vi "Serial_read.vi"() -> ()   [LabVIEW 2016]
uses:
  Program Files (x86)/National Instruments/LabVIEW 2016/examples/Instrument IO/Serial/support/Serial - Settings.ctl
  Program Files (x86)/National Instruments/LabVIEW 2016/examples/Instrument IO/Serial/support/Serial - XON-XOFF Characters.ctl
  Program Files (x86)/National Instruments/LabVIEW 2016/examples/Instrument IO/Serial/support/Serial - ASCII Characters.ctl
  <vilib>/Instr/_visa.llb/VISA Configure Serial Port (Instr).vi
  <vilib>/Utility/file.llb/Write Delimited Spreadsheet (DBL).vi
panel:
  out "element":dbl
  out "error out":errorcluster
  out "Serial Settings:Number of Bytes at Serial Port":u32
  out "Byte array has been sent":u8[](array[numeric])
  in  "Payload  Byte to be sent":u8[](array[numeric])
  in  "Type of Message to be sent":T1(ring)
  in  "MCU Address to be sent":string(combo)
  in  "Save":bool
  out "Waveform Chart 2":dbl(graph)
  out "Thermometer":dbl(slide) scale=0.0..100.0
  out "Waveform Chart":dynamicdata(graph)
  out "Extracted Numbers":dbl[](array[numeric]) format="%#.6g"
  in  "Stop":bool
  out "String":string
  in  "Termination Character":u8=10 format="%.0x"
  in  "End Write on Termination Character?":bool=TRUE
  in  "VISA resource name":refnum<visa-resource-name>="COM1"
  in  "XON/XOFF Characters":T2={"XON"=enum."DC1", "XOFF"=enum."DC3"}
  in  "Serial Settings":T4={"baud rate"=9600, "data bits"=8, "parity"=enum."None", "stop bits"=10, "flow control"=0} {"flow control" items=["None"=0, "XON/XOFF"=1, "RTS/CTS"=2, "DTR/DSR"=4]; "stop bits" items=["1.0"=10, "1.5"=15, "2.0"=20]; "data bits" min=5 max=8 step=1; "baud rate" items=["75"=75, "110"=110, "134"=134, "150"=150, "300"=300, "600"=600, "1200"=1200, "1800"=1800, "2400"=2400, "4800"=4800, "7200"=7200, "9600"=9600, "14400"=14400, "19200"=19200, "28800"=28800, "38400"=38400, "56000"=56000, "57600"=57600, "115200"=115200, "128000"=128000, "230400"=230400]}
  in  "End Read on Termination Character?":bool=TRUE
  out "Response":string
  in  "Read Count":u32=1000
  in  "Read":bool
  in  "Write":bool
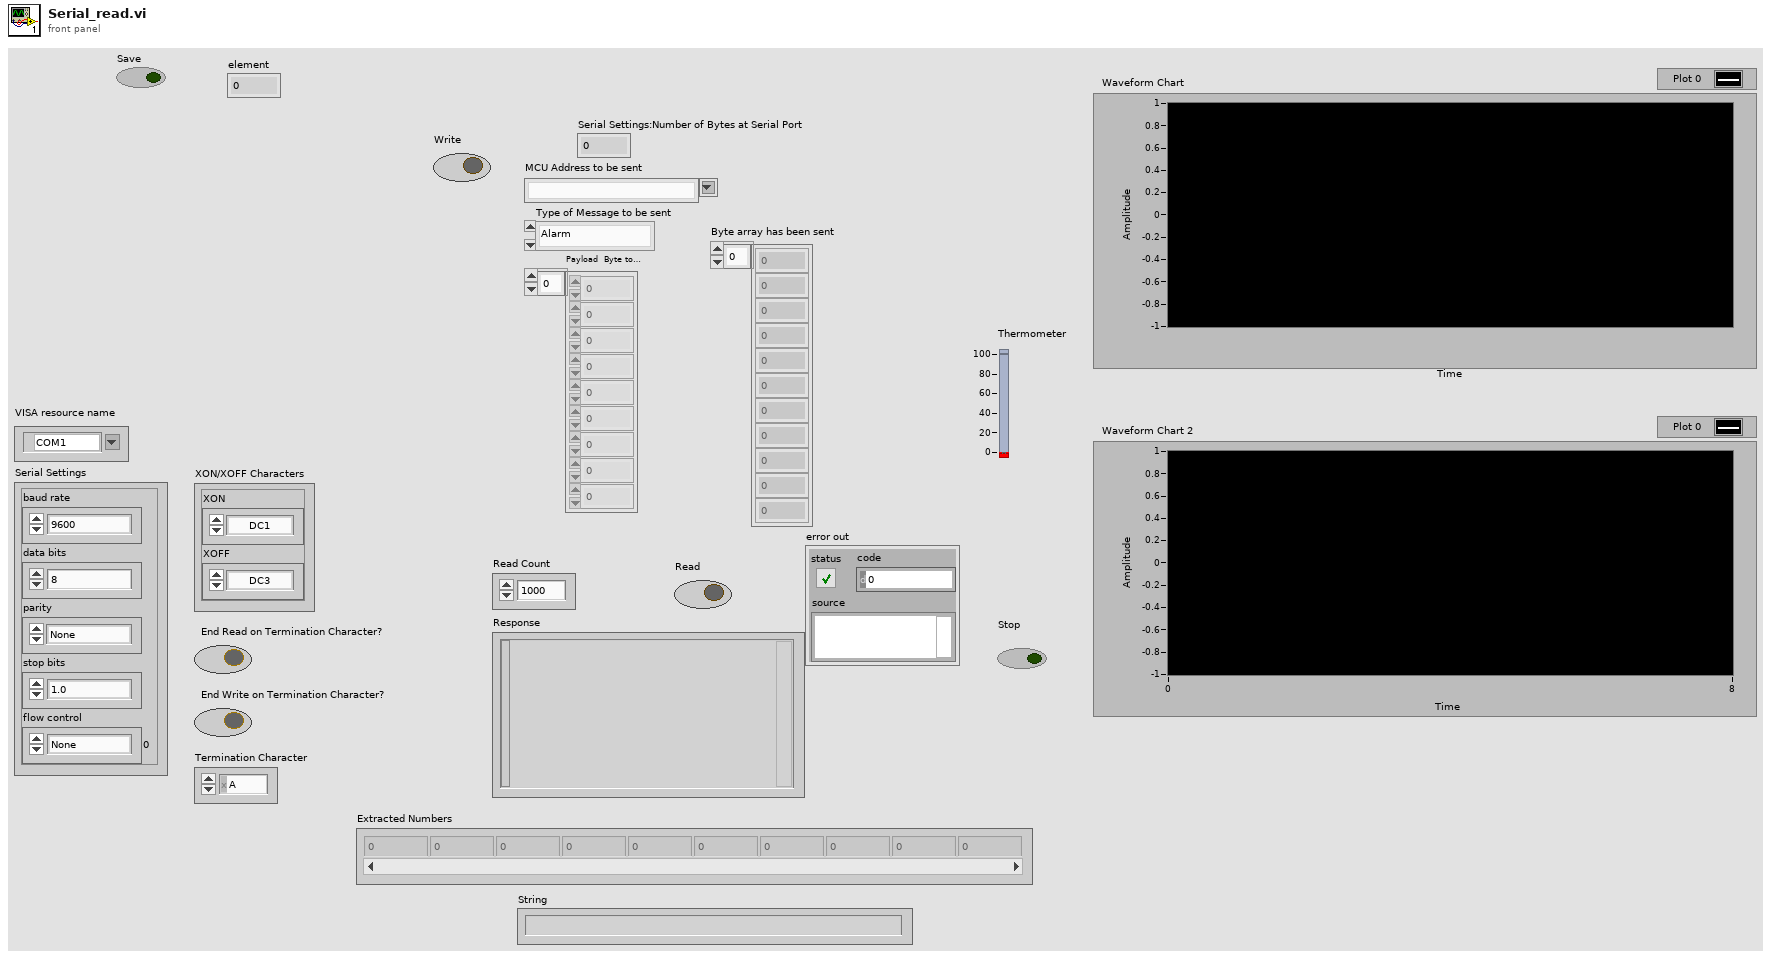
[diagram p1: front panel]
types:
  T1 = enum8{"Alarm", "Error", "Time and date", "Status", "Request"}
  T2 = typedef "Serial - XON-XOFF Characters.ctl" = cluster{"XON":T3, "XOFF":T3}
  T3 = typedef "Serial - ASCII Characters.ctl" = enum16{"NUL", "SOH", "STX", "ETX", "EOT", "ENQ", "ACK", "BEL", "BS", "HT", "LF", "VT", "FF", "CR", "SO", "SI", "DLE", "DC1", "DC2", "DC3", "DC4", "NAK", "SYN", "ETB", "CAN", "EM", "SUB", "ESC", "FS", "GS", "RS", "US", "SP", "!", "\"", "#", "$", "%", "&", "'", "(", ")", "*", "+", ",", "- (-)", ".", "/", "0", "1", "2", "3", "4", "5", "6", "7", "8", "9", ":", ";", "<", "=", ">", "?", "@", "A", "B", "C", "D", "E", "F", "G", "H", "I", "J", "K", "L", "M", "N", "O", "P", "Q", "R", "S", "T", "U", "V", "W", "X", "Y", "Z", "[", "\\", "]", "^", "_", "`", "a", "b", "c", "d", "e", "f", "g", "h", "i", "j", "k", "l", "m", "n", "o", "p", "q", "r", "s", "t", "u", "v", "w", "x", "y", "z", "{", "|", "}", "~"}
  T4 = typedef "Serial - Settings.ctl" = cluster{"baud rate":u32, "data bits":u16, "parity":enum16{"None", "Odd", "Even", "Mark", "Space"}, "stop bits":u16, "flow control":u16}
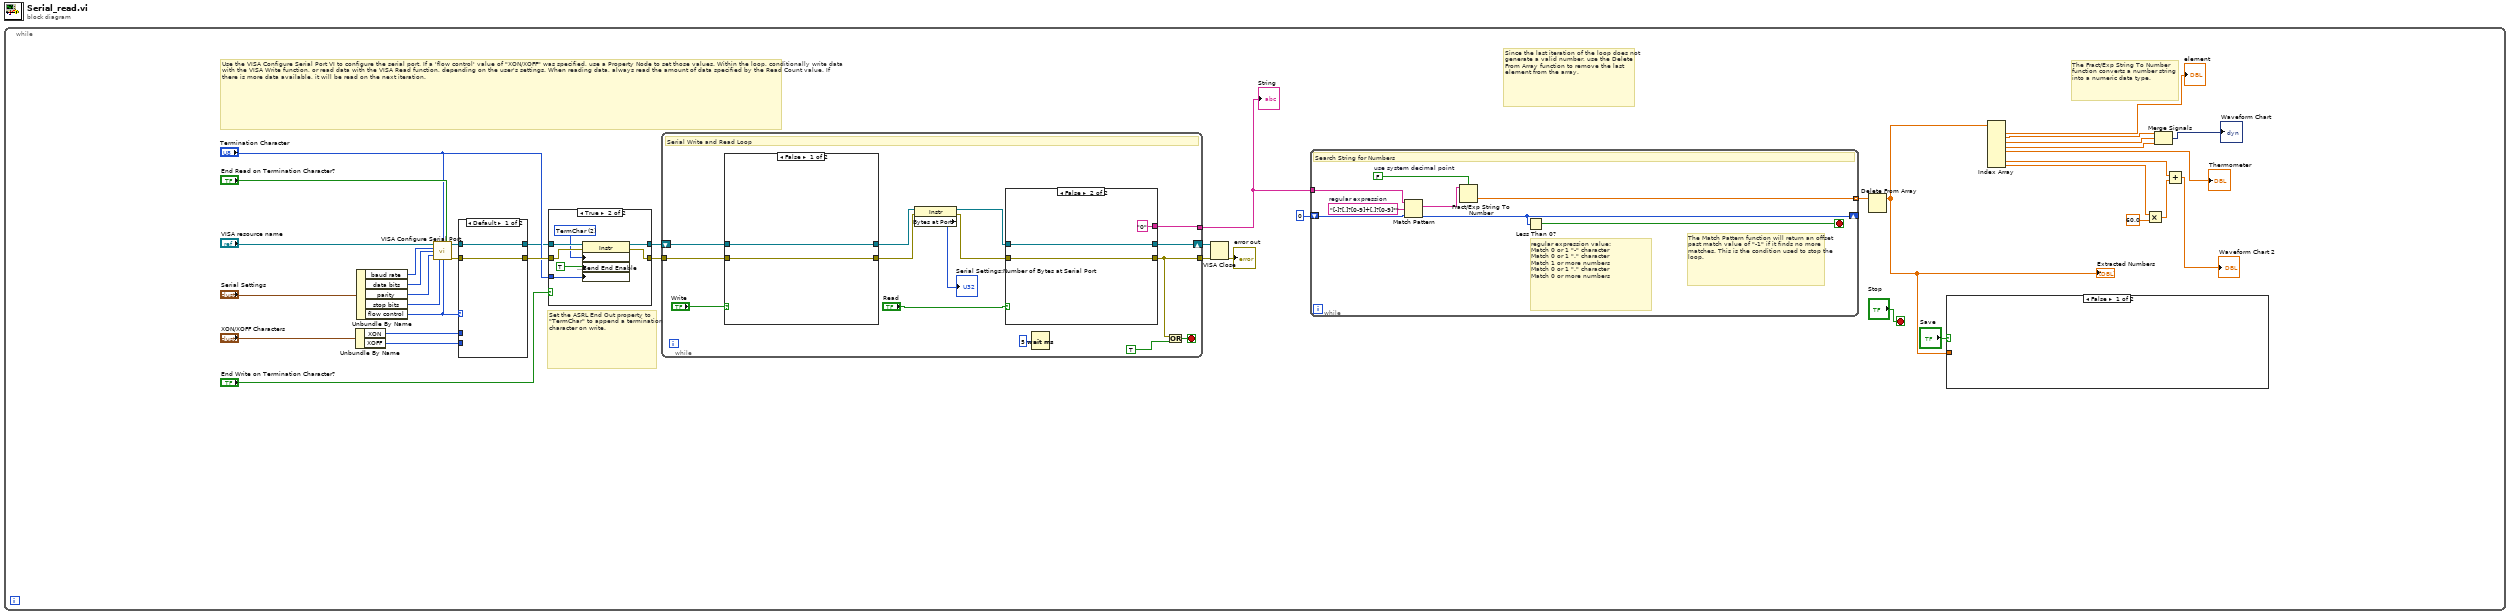
[diagram p0: block diagram]
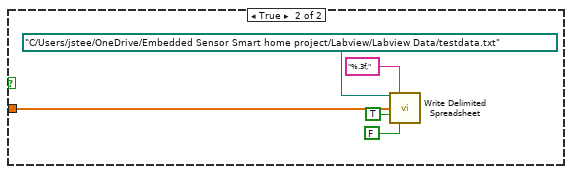
[diagram p2: hidden frame]
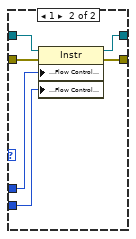
[diagram p4: hidden frame]
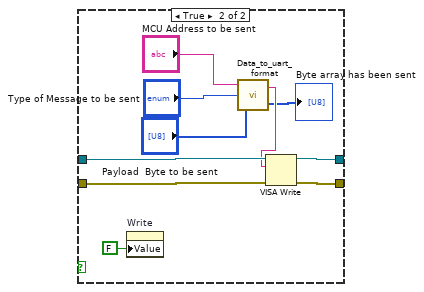
[diagram p5: hidden frame]
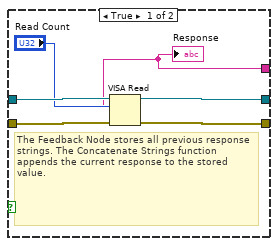
[diagram p6: hidden frame]
diagram:
  n1 = while {
    stop <- "Stop" stop-if-true
    # "The Fract/Exp String To Number function converts a number string into a numeric data type."
    # "Since the last iteration of the loop does not generate a valid number, use the Delete From Array function to remove the last element from the array."
    # "Set the ASRL End Out property to \"TermChar\" to append a termination character on write."
    # "Use the VISA Configure Serial Port VI to configure the serial port. If a 'flow control' value of \"XON/XOFF\" was specified, use a Property Node to set those values. Within the loop, conditionally write data with the VISA Write function, or read data with the VISA Read function, depending on the user's settings. When reading data, always read the amount of data specified by the Read Count value. If there is more data available, it will be read on the next iteration."
    n2 = Unbundle By Name("XON/XOFF Characters") -> ("XON"=w26:T3, "XOFF"=w25:T3)
    n3 = Unbundle By Name("Serial Settings") -> ("baud rate"=w32:u32, "data bits"=w33:u16, "parity"=w34:enum16{"None", "Odd", "Even", "Mark", "Space"}, "stop bits"=w35:u16, "flow control"=w27:u16)
    n4 = call-poly "VISA Configure Serial Port"("VISA resource name"="VISA resource name", "termination char\n(0xA = '\\n' = LF)"="Termination Character", "Enable Termination\nChar (T)"="End Read on Termination Character?", "baud rate (9600)"=w32, "data bits (8)"=w33, "parity (0:none)"=w34, "stop bits (10: 1 bit)"=w35, "flow control (0:none)"=w27) -> ("VISA resource name out"=w36:refnum<visa-resource-name>, "error out"=w37:errorcluster)  [unwired: 2 in, 4 out]
    n5 = case shown="Default" w27 {
      tunnel: [w62 w69] -> w24
      tunnel: [w63 w68] -> w4
      tunnel: w37 -> [w62 w67]
      tunnel: w36 -> [w63 w66]
      tunnel: w26 -> [_ w65]
      tunnel: w25 -> [_ w64]
      frame Default {
      }
      frame 1 {
        n6 = property class="Instr"(reference=w66, error in=w67, "Serial Settings:Flow Control XON Character"=w65, "Serial Settings:Flow Control XOFF Character"=w64) -> (reference out=w68:refnum<visa-resource-name>, error out=w69:errorcluster)
      }
    }
    n7 = case shown="True" "End Write on Termination Character?" {
      tunnel: w4 -> [w53 w61]
      tunnel: w24 -> [w54 w60]
      tunnel: [w53 w59] -> w22
      tunnel: [w54 w58] -> w23
      tunnel: "Termination Character" -> [_ w56]
      frame False {
      }
      frame True {
        w57 = u16 2 items=["None", "LastBit", "TermChar", "Break"] ("Serial Settings:Serial End Mode for Writes")
        n8 = property class="Instr"(reference=w61, error in=w60, "Serial Settings:End Mode for Writes"=w57, "Message Based Settings:Send End Enable"=TRUE, "Message Based Settings:Termination Character"=w56) -> (reference out=w59:refnum<visa-resource-name>, error out=w58:errorcluster)
      }
    }
    n9 = while {
      shift-right: [w84] -> w28
      shift-left: w22 -> [w83]
      tunnel: w23 -> [w82]
      tunnel: [w79] -> w29
      tunnel: [w76] -> w17
      stop <- w80 stop-if-true
      # "Serial Write and Read Loop"
      n10 = case shown="False" "Write" {
        tunnel: w83 -> [w86 w96]
        tunnel: w82 -> [w85 w95]
        tunnel: [w86 w94] -> w75
        tunnel: [w85 w93] -> w71
        frame False {
        }
        frame True {
          n11 = property on="Write" class="Bool (strict)"("Value"=FALSE ("Write")) -> ()  [unwired: 2 in, 2 out]
          n12 = call "Data_to_uart_format.vi"("Payload  Byte to be sent"="Payload  Byte to be sent", "Type of Message to be sent"="Type of Message to be sent", "MCU Address to be sent"="MCU Address to be sent") -> ("Byte array has been sent"=→"Byte array has been sent":u8[], "Converted Message"=w88:string)
          n13 = VISA Write(VISA resource name=w96, write buffer=w88, error in (no error)=w95) -> (VISA resource name out=w94:refnum<visa-resource-name>, error out=w93:errorcluster)  [unwired: 1 out]
        }
      }
      n14 = property class="Instr"(reference=w75, error in=w71) -> (reference out=w72:refnum<visa-resource-name>, error out=w70:errorcluster, "Bytes at Port"=→"Serial Settings:Number of Bytes at Serial Port":u32)
      n15 = case shown="False" "Read" {
        tunnel: [w100 w105] -> w84
        tunnel: w72 -> [w102 w105]
        tunnel: [w98 w104] -> w79
        tunnel: w70 -> [w101 w104]
        tunnel: [w97 "0"] -> w76
        frame True {
          # "The Feedback Node stores all previous response strings. The Concatenate Strings function appends the current response to the stored value."
          n16 = VISA Read(VISA resource name=w102, byte count="Read Count", error in (no error)=w101) -> (VISA resource name out=w100:refnum<visa-resource-name>, read buffer=w97:string, error out=w98:errorcluster)  [unwired: 1 out]
          "Response" <- w97
        }
        frame False {
        }
      }
      n17 = Wait (ms)(milliseconds to wait=u32 5) -> ()  [unwired: 1 out]
      n18 = Or(x=w79, y=TRUE ("Stop")) -> (x .or. y?=w80:bool)
    }
    "String" <- w17
    n19 = VISA Close(VISA resource name=w28, error in (no error)=w29) -> (error out=→"error out":errorcluster)
    n20 = while {
      tunnel: w17 -> [w52]
      shift-left: 0 -> [w50]
      shift-right: [w47] -> _
      tunnel: [w45] -> w7 mode=indexing
      stop <- w51 stop-if-true
      w49 = FALSE  # use system decimal point
      w46 = "[-]?[.]?[0-9]+[.]?[0-9]*"  # regular expression
      # "The Match Pattern function will return an offset past match value of \"-1\" if it finds no more matches. This is the condition used to stop the loop."
      # "regular expression value:\nMatch 0 or 1 \"-\" character\nMatch 0 or 1 \".\" character\nMatch 1 or more numbers\nMatch 0 or 1 \".\" character\nMatch 0 or more numbers"
      # "Search String for Numbers"
      n21 = Match Pattern(string=w52, regular expression=w46, offset (0)=w50) -> (match substring=w48:string, offset past match=w47:i32)  [unwired: 2 out]
      n22 = Fract/Exp String To Number(use system decimal point (T)=w49, string=w48) -> (number=w45:dbl)  [unwired: 2 in, 1 out]
      n23 = Less Than 0?(x=w47) -> (x < 0?=w51:bool)
    }
    n24 = Delete From Array(array=w7) -> (array with subset deleted=w6:dbl[])  [unwired: 2 in, 1 out]
    "Extracted Numbers" <- w6
    n25 = case shown="False" "Save" {
      tunnel: w6 -> [_ w40]
      frame False {
      }
      frame True {
        n26 = call-poly <vilib>:"Write Delimited Spreadsheet.vi"("file path (dialog if empty)"=path "C:/Users/jstee/OneDrive/Embedded Sensor Smart home project/Labview/Labview Data/testdata.txt", "format (%.3f)"="%.3f,", "1D data"=w40, "append to file? (new file:F)"=TRUE, "transpose? (no:F)"=FALSE) -> ()  [unwired: 9 in, 2 out]
      }
    }
    n27 = Index Array(array=w6) -> (element #1=→"element":dbl, element #2=w16:dbl, element #3=w15:dbl, element #4=w2:dbl, element #5=→"Thermometer":dbl, element #7=w13:dbl, element #8=w11:dbl)  [unwired: 8 in, 1 out]
    n28 = Multiply(x=w11, y=60.0) -> (x*y=w12:dbl)
    n29 = Merge Signals(w16, w15, w2) -> (→"Waveform Chart":dynamicdata)
    n30 = Add(x=w13, y=w12) -> (x+y=→"Waveform Chart 2":dbl)
  }
